vi "SetFlapsState.vi"(8 "error in":errorcluster, 11 "FlapsState":enum16{"In", "Out"}(ring)) -> (0 "error out":errorcluster)   [LabVIEW 2016]
uses:
  Robot Global Data.vi
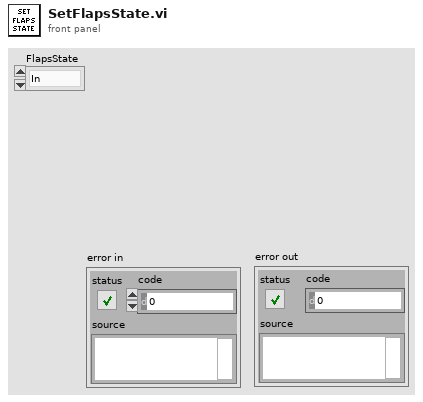
[diagram p1: front panel]
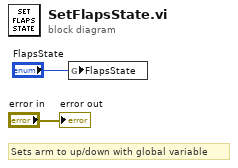
[diagram p0: block diagram]
diagram:
  # "Sets arm to up/down with global variable"
  n1 = global write "Robot Global Data.vi" "FlapsState"("FlapsState") -> ()
  "error out" <- "error in"
